vi "Global banco.vi"() -> ()   [LabVIEW 2019]
panel:
  in  "banco":i8
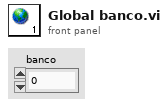
[diagram p1: front panel]
diagram:
